vi "PH_Beamline_Common.set Crosshair.vi"(2 "CtlRef":refnum<vi>, 3 "State":i16, 4 "no link":bool, 5 "error in (no error)":errorcluster) -> (19 "error out":errorcluster)   [LabVIEW 2014, in "PH_Beamline_Common.lvlib"]
uses:
  PH_Beamline_Common.lvlib
  PH_Common/PH_Common.lvlib
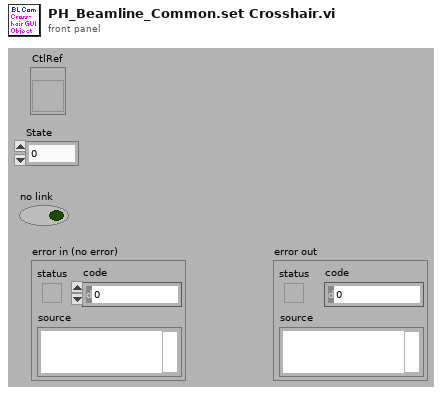
[diagram p1: front panel]
types:
  T1 = cluster{"Width":i16, "Style":enum32{"Solid", "Dash", "Dot", "DashDot", "DashDotDot"}}
  T2 = cluster{"left":i16, "top":i16, "right":i16, "bottom":i16}
  T3 = cluster{"Width":u16, "Style":enum32{"Solid", "Dash", "Dot", "DashDot", "DashDotDot"}}
  T4 = cluster{"left":i32, "top":i32, "right":i32, "bottom":i32}
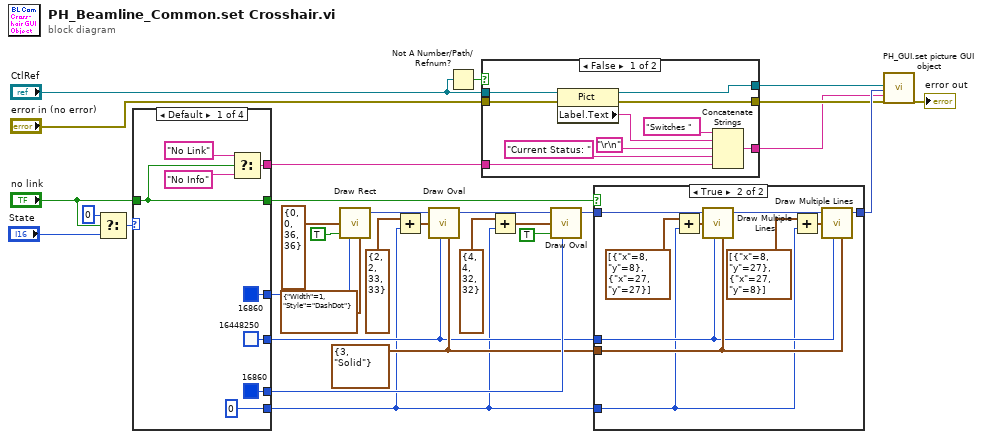
[diagram p0: block diagram]
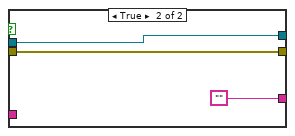
[diagram p2: hidden frame]
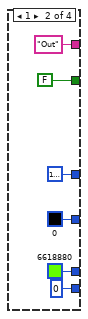
[diagram p4: hidden frame]
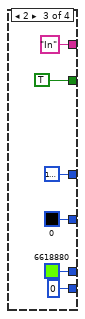
[diagram p5: hidden frame]
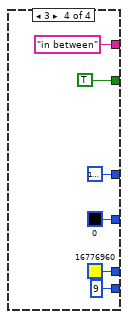
[diagram p6: hidden frame]
diagram:
  w17 = T3 {"Width"=3, "Style"=enum."Solid"} ("pen")
  n1 = Select(t=i16 0, s="no link", f="State") -> (s? t:f=w14:i16)
  n2 = case shown="Default" w14 {
    tunnel: [u32 16860 u32 6618880 u32 6618880 u32 16776960] -> w23
    tunnel: [u32 16860 u32 16777216 u32 16777216 u32 16777216] -> w24
    tunnel: [u32 16448250 u32 0 u32 0 u32 0] -> w16
    tunnel: "no link" -> [w32 _ _ _]
    tunnel: [w33 "Out" "In" "in between"] -> w13
    tunnel: [w32 FALSE ("no link") TRUE ("no link") TRUE ("no link")] -> w12
    tunnel: [0 ("x") 0 ("x") 0 ("x") 9 ("x")] -> w7
    frame Default {
      n3 = Select(t="No Link", s=w32, f="No Info") -> (s? t:f=w33:string)
    }
    frame 1 {
    }
    frame 2 {
    }
    frame 3 {
    }
  }
  n4 = call <vilib>:"Draw Rect.vi"("rect"=T2 {"left"=0, "top"=0, "right"=36, "bottom"=36}, "fill?(F)"=TRUE, "color(black)"=w24, "pen"=T1 {"Width"=1, "Style"=enum."DashDot"}) -> ("new picture"=w19:picture)  [unwired: 5 in]
  n5 = Add(x=T2 {"left"=2, "top"=2, "right"=33, "bottom"=33} ("rect"), y=w7) -> (x+y=w8:T4)
  n6 = call <vilib>:"Draw Oval.vi"("picture"=w19, "rect"=w8, "color(black)"=w16, "pen"=w17) -> ("new picture"=w21:picture)  [unwired: 5 in]
  n7 = Not A Number/Path/Refnum?(number/path/refnum="CtlRef") -> (NaN/Path/Refnum?=w2:bool)
  n8 = case shown="False" w2 {
    tunnel: "CtlRef" -> [w62 w69]
    tunnel: "error in (no error)" -> [w61 w68]
    tunnel: w13 -> [w60 _]
    tunnel: [w59 w69] -> w5
    tunnel: [w58 w68] -> w4
    tunnel: [w57 ""] -> w3
    frame False {
      n9 = property class="Pict"(reference=w62, error in=w61) -> (reference out=w59:refnum<vi>, error out=w58:errorcluster, "Label.Text"=w65:string)
      n10 = Concatenate Strings("Switches " ("string"), w65, "\r\n", "Current Status: " ("string"), w60) -> (w57:string)
    }
    frame True {
    }
  }
  n11 = Add(x=T2 {"left"=4, "top"=4, "right"=32, "bottom"=32} ("rect"), y=w7) -> (x+y=w11:T4)
  n12 = call <vilib>:"Draw Oval.vi"("picture"=w21, "rect"=w11, "fill?(F)"=TRUE, "color(black)"=w23) -> ("new picture"=w18:picture)  [unwired: 5 in]
  n13 = case shown="True" w12 {
    tunnel: w18 -> [w70 w80]
    tunnel: w17 -> [_ w78]
    tunnel: w16 -> [_ w77]
    tunnel: [w70 w76] -> w6
    tunnel: w7 -> [_ w71]
    frame False {
    }
    frame True {
      n14 = Add(x=cluster{"x":i16, "y":i16}[] [{"x"=8, "y"=8}, {"x"=27, "y"=27}] ("line endpoints"), y=w71) -> (x+y=w74:cluster{"x":i32, "y":i32}[])
      n15 = call <vilib>:"Draw Multiple Lines.vi"("picture"=w80, "line endpoints"=w74, "color(black)"=w77, "pen"=w78) -> ("new picture"=w79:picture)  [unwired: 5 in]
      n16 = Add(x=cluster{"x":i16, "y":i16}[] [{"x"=8, "y"=27}, {"x"=27, "y"=8}] ("line endpoints"), y=w71) -> (x+y=w72:cluster{"x":i32, "y":i32}[])
      n17 = call <vilib>:"Draw Multiple Lines.vi"("picture"=w79, "line endpoints"=w72, "color(black)"=w77, "pen"=w78) -> ("new picture"=w76:picture)  [unwired: 5 in]
    }
  }
  n18 = call "PH_GUI.set picture GUI object.vi"("CtlRef"=w5, "Picture"=w6, "Tip Strip (\"\")"=w3, "error in (no error)"=w4) -> ("error out"=→"error out":errorcluster)  [unwired: 15 in]
